vi "Set Screenpop Loop References.vi"(7 "Data Loop Data in":T1, 8 "error in":errorcluster, 11 "call chain":string[](array[string])) -> (0 "error out":errorcluster, 2 "Data Loop Data out":T1)   [LabVIEW 2018]
uses:
  Type Defs/Screenpop Loop Data.ctl
  Support/Message Queue/Message Cluster.ctl
  Support/Message Queue/Message Queue.lvlib
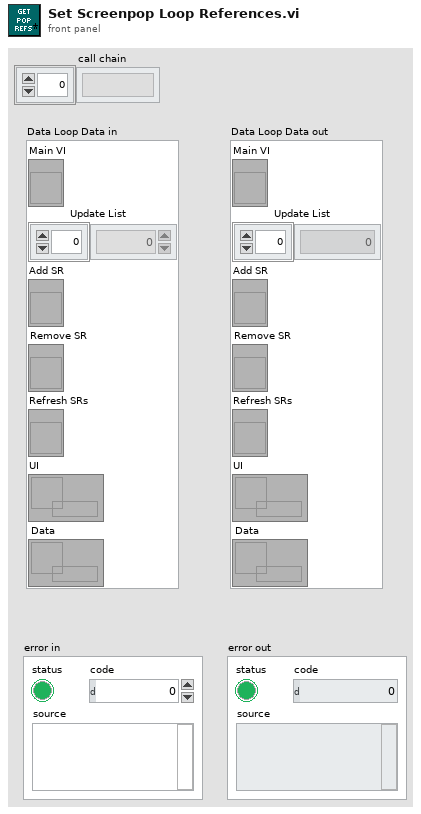
[diagram p1: front panel]
types:
  T1 = typedef "Screenpop Loop Data.ctl" = cluster{"Main VI":refnum<vi>, "Update List":i32[], "Add SR":refnum<vi>, "Remove SR":refnum<vi>, "Refresh SRs":refnum<vi>, "UI":refnum<queue>, "Data":refnum<queue>}
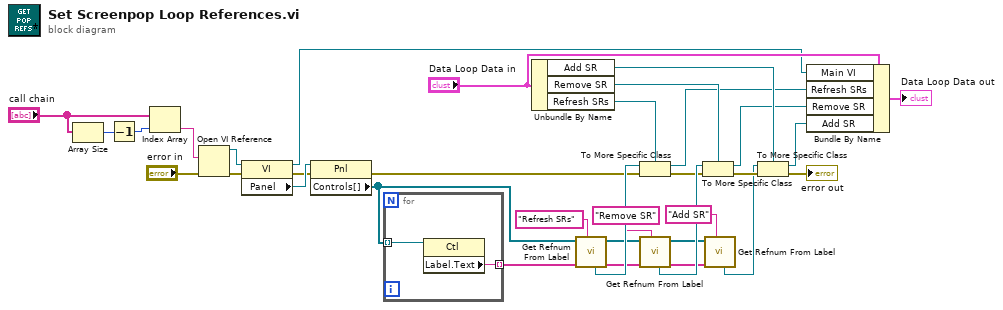
[diagram p0: block diagram]
diagram:
  n1 = Array Size(array="call chain") -> (size(s)=w18:i32)
  n2 = Decrement(x=w18) -> (x-1=w19:i32)
  n3 = Index Array(array="call chain", index=w19) -> (element=w20:string)
  n4 = Open VI Reference(vi path=w20, error in (no error)="error in") -> (vi reference=w33:refnum<vi>, error out=w28:errorcluster)  [unwired: 4 in]
  n5 = property class="VI"(reference=w33, error in=w28) -> (reference out=w16:refnum<vi>, error out=w29:errorcluster, "Panel"=w30:refnum<vi>)
  n6 = property class="Pnl"(reference=w30, error in=w29) -> (error out=w13:errorcluster, "Controls[]"=w21:refnum<vi>[])  [unwired: 1 out]
  n7 = for {
    tunnel: w21 -> [w36] mode=indexing
    tunnel: [w35] -> w22 mode=indexing
    n8 = property class="Ctl"(reference=w36) -> ("Label.Text"=w35:string)  [unwired: 1 in, 2 out]
  }
  n9 = Unbundle By Name("Data Loop Data in") -> ("Add SR"=w7:refnum<vi>, "Remove SR"=w5:refnum<vi>, "Refresh SRs"=w6:refnum<vi>)
  n10 = call "Get Refnum From Label.vi"("label"="Refresh SRs", "label array in"=w22, "controls[] in"=w21) -> ("label array out"=w24:string[], "controls[] out"=w23:refnum<vi>[], "refnum out"=w25:refnum<vi>)  [unwired: 6 in]
  n11 = To More Specific Class(target class=w6, reference=w25, error in=w13) -> (specific class reference=w3:refnum<vi>, error out=w26:errorcluster)
  n12 = call "Get Refnum From Label.vi"("label"="Remove SR", "label array in"=w24, "controls[] in"=w23) -> ("label array out"=w11:string[], "controls[] out"=w12:refnum<vi>[], "refnum out"=w27:refnum<vi>)  [unwired: 6 in]
  n13 = To More Specific Class(target class=w5, reference=w27, error in=w26) -> (specific class reference=w4:refnum<vi>, error out=w15:errorcluster)
  n14 = call "Get Refnum From Label.vi"("label"="Add SR", "label array in"=w11, "controls[] in"=w12) -> ("refnum out"=w8:refnum<vi>)  [unwired: 6 in, 2 out]
  n15 = To More Specific Class(target class=w7, reference=w8, error in=w15) -> (specific class reference=w9:refnum<vi>, error out=→"error out":errorcluster)
  n16 = Bundle By Name(cluster="Data Loop Data in", "Main VI"=w16, "Refresh SRs"=w3, "Remove SR"=w4, "Add SR"=w9) -> (→"Data Loop Data out":T1)
